vi "Construct Buffered Log Sink.vi"(9 "Buffer Size (128)":i32=128, 10 "Buffer Timeout ms (-1)":i32=-1, 11 "Sink to Buffer":refnum<class "Log Sink.lvclass">) -> (3 "Buffered Log Sink out":refnum<class "Buffered Log Sink.lvclass">)   [LabVIEW 2019, in "Buffered Log Sink.lvclass"]
doc: "Create a buffered sink - inject another sink type to add buffering to that sink type. This is useful for any sink type where writes occur a lot of overhead, like writing to a database. Log events will be passed from the buffer when a timeout occurs, or when the buffer size is met. Any un logged events will be passed to the destination sink on shutdown."
uses:
  <vilib>/gpm_packages/@cs/event-logger/Source/Buffered Log Sink/Buffered Log Sink.lvclass
  <vilib>/gpm_packages/@cs/event-logger/Source/Composed Log/Log Sink/Log Sink.lvclass
  <vilib>/gpm_packages/@cs/event-logger/Source/Buffered Log Sink/Buffered Log Sink.lvclass/Buffered Log Sink.ctl
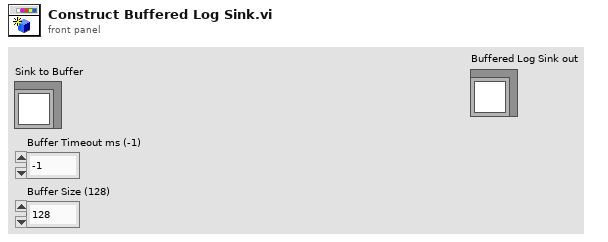
[diagram p1: front panel]
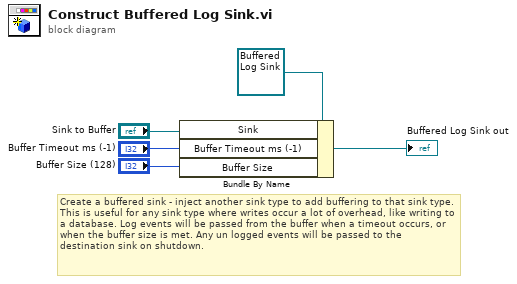
[diagram p0: block diagram]
diagram:
  # "Create a buffered sink - inject another sink type to add buffering to that sink type. This is useful for any sink type where writes occur a lot of overhead, like writing to a database. Log events will be passed from the buffer when a timeout occurs, or when the buffer size is met. Any un logged events will be passed to the destination sink on shutdown."
  n1 = Bundle By Name(cluster=refnum<class "Buffered Log Sink.lvclass"> refnum ("Buffered Log Sink in"), "Sink"="Sink to Buffer", "Buffer Timeout ms (-1)"="Buffer Timeout ms (-1)", "Buffer Size"="Buffer Size (128)") -> (→"Buffered Log Sink out":refnum<class "Buffered Log Sink.lvclass">)
